vi "Query Reference Frequency.vi"(8 "error in (no error)":errorcluster, 11 "VISA resource name":refnum<visa-resource-name>="COM1") -> (0 "error out":errorcluster, 2 "Frequency output":string, 3 "VISA resource name out":refnum<visa-resource-name>)   [LabVIEW 2017]
panel:
  out "read buffer":string
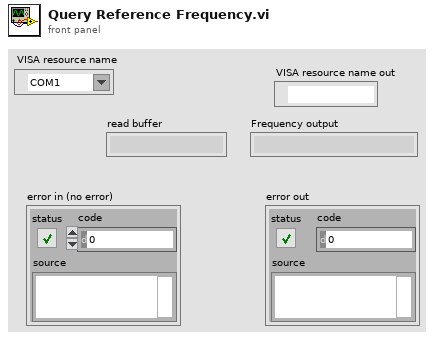
[diagram p1: front panel]
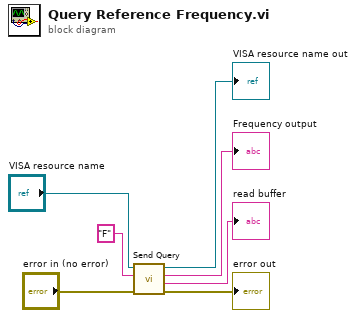
[diagram p0: block diagram]
diagram:
  n1 = call "Send Query.vi"("error in (no error)"="error in (no error)", "query string"="F", "VISA resource name"="VISA resource name") -> ("error out"=→"error out":errorcluster, "read buffer"=→"read buffer":string, "query output"=→"Frequency output":string, "VISA resource name out"=→"VISA resource name out":refnum<visa-resource-name>)  [unwired: 5 in]
